vi "Rearrange Array 2D DBL.vi"(4 "Index Map":i32[](array[numeric]), 6 "Array":dbl[][](array[numeric])) -> (2 "Rearranged Array":dbl[][](array[numeric]))   [LabVIEW 2013]
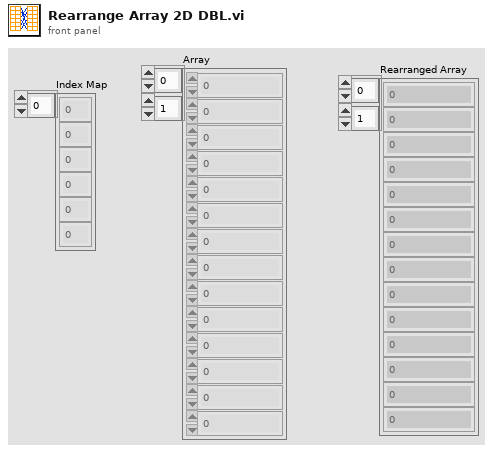
[diagram p1: front panel]
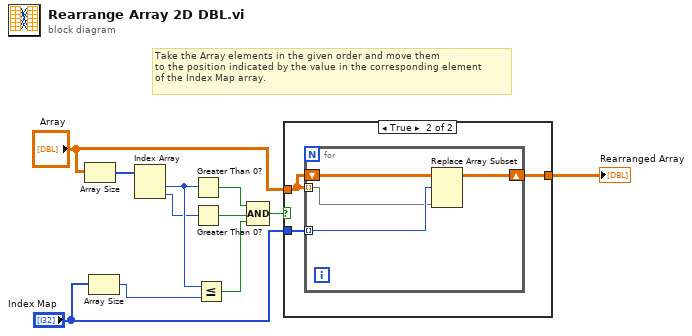
[diagram p0: block diagram]
diagram:
  # "Take the Array elements in the given order and move them\nto the position indicated by the value in the corresponding element\nof the Index Map array."
  n1 = Array Size(array="Array") -> (size(s)=w8:i32[])
  n2 = Array Size(array="Index Map") -> (size(s)=w1:i32)
  n3 = Index Array(array=w8) -> (element #1=w7:i32, element #2=w4:i32)  [unwired: 2 in]
  n4 = Greater Than 0?(x=w7) -> (x > 0?=w5:bool)
  n5 = Greater Than 0?(x=w4) -> (x > 0?=w3:bool)
  n6 = Less Or Equal?(x=w7, y=w1) -> (x <= y?=w2:bool)
  n7 = Compound Arithmetic op=AND(w5, w3, w2) -> (w6:bool)
  n8 = case shown="True" w6 {
    tunnel: "Index Map" -> [_ w15]
    tunnel: "Array" -> [w12 w13]
    tunnel: [w12 w14] -> w11
    frame False {
    }
    frame True {
      n9 = for {
        tunnel: w15 -> [w17] mode=indexing
        shift-right: [w18] -> w14
        shift-left: w13 -> [w19]
        tunnel: w13 -> [w16] mode=indexing
        n10 = Replace Array Subset(array=w19, new element=w16, index (row)=w17) -> (w18:dbl[][])  [unwired: 1 in]
      }
    }
  }
  "Rearranged Array" <- w11
